vi "ShiftLeft (SubVI).vi"(11 "Array in":i32[](array[numeric])=[0, 3, 2, 1]) -> (2 "tiles moved?":bool, 3 "Array out":i32[](array[numeric])=[0, 3, 2, 1])   [LabVIEW 2020]
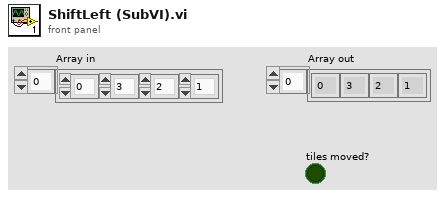
[diagram p1: front panel]
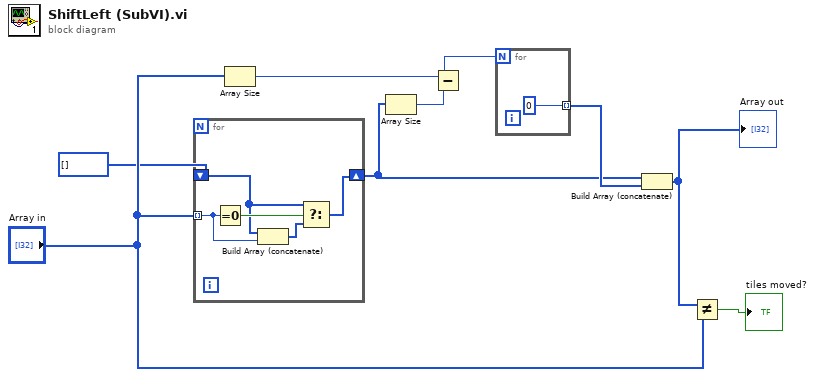
[diagram p0: block diagram]
diagram:
  n1 = for {
    tunnel: "Array in" -> [w12] mode=indexing
    shift-right: [w13] -> w4
    shift-left: i32[] [] ("Array") -> [w10]
    n2 = Equal To 0?(x=w12) -> (x = 0?=w14:bool)
    n3 = Build Array (concatenate)(w10, w12) -> (w11:i32[])
    n4 = Select(t=w10, s=w14, f=w11) -> (s? t:f=w13:i32[])
  }
  n5 = Array Size(array="Array in") -> (size(s)=w3:i32)
  n6 = Array Size(array=w4) -> (size(s)=w2:i32)
  n7 = Subtract(x=w3, y=w2) -> (x-y=w6:i32)
  n8 = for {
    N: w6 -> [_]
    tunnel: [0 ("Numeric")] -> w5 mode=indexing
  }
  n9 = Build Array (concatenate)(w4, w5) -> (w7:i32[])
  "Array out" <- w7
  n10 = Not Equal?(x=w7, y="Array in") -> (x != y?=→"tiles moved?":bool)
